vi "Ramped Deadband.vi"(3 "End of Ramp down":dbl=0.2 format="%#_13g", 4 "Beginning of Ramp Down":dbl=0.5 format="%#_13g", 5 "Error Value In":dbl) -> (2 "Error Value out":dbl)   [LabVIEW 2020]
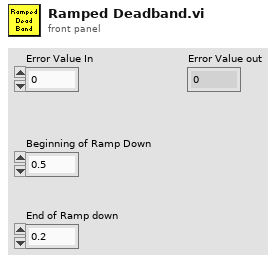
[diagram p1: front panel]
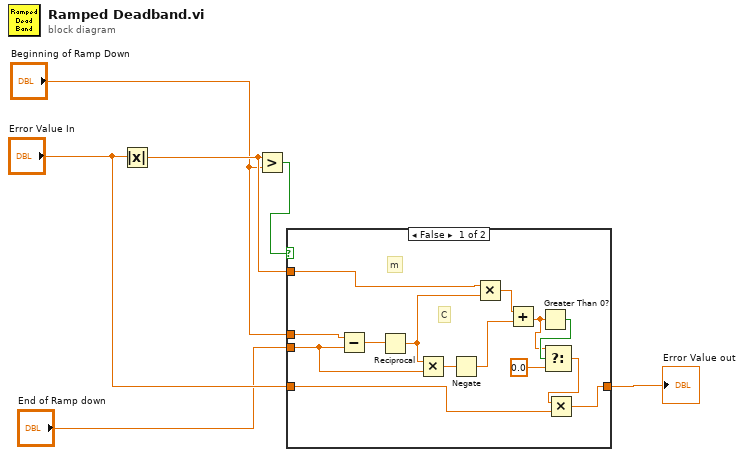
[diagram p0: block diagram]
diagram:
  n1 = Absolute Value(x="Error Value In") -> (abs(x)=w6:dbl)
  n2 = Greater?(x=w6, y="Beginning of Ramp Down") -> (0:w1:bool)
  n3 = case shown="False" w1 {
    tunnel: [w9 w21] -> w2
    tunnel: "Error Value In" -> [w7 w21]
    tunnel: "Beginning of Ramp Down" -> [w20 _]
    tunnel: "End of Ramp down" -> [w18 _]
    tunnel: w6 -> [w15 _]
    frame False {
      # "C"
      # "m"
      n4 = Subtract(x=w20, y=w18) -> (x-y=w19:dbl)
      n5 = Reciprocal(x=w19) -> (1/x=w16:dbl)
      n6 = Multiply(x=w16, y=w18) -> (x*y=w17:dbl)
      n7 = Negate(x=w17) -> (-x=w13:dbl)
      n8 = Multiply(x=w15, y=w16) -> (x*y=w14:dbl)
      n9 = Add(x=w14, y=w13) -> (x+y=w11:dbl)
      n10 = Greater Than 0?(x=w11) -> (x > 0?=w12:bool)
      n11 = Select(t=w11, s=w12, f=0.0) -> (s? t:f=w8:dbl)
      n12 = Multiply(x=w8, y=w7) -> (x*y=w9:dbl)
    }
    frame True {
    }
  }
  "Error Value out" <- w2
